vi "Load.vi"(8 "error in (no error)":errorcluster, 11 "Data File":path) -> (0 "error out":errorcluster, 3 "dup Data File":path)   [LabVIEW 2014, in "Map Data.lvlib"]
doc: "Loads data into the address book data store from a file on disk. If the file does not exist, the data store is initialized to being empty."
uses:
  Map Data.lvlib
  MapCommand.ctl
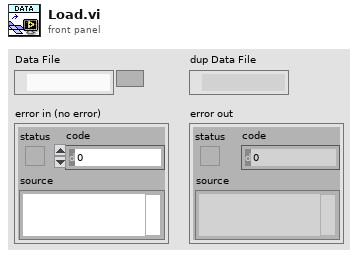
[diagram p1: front panel]
types:
  T1 = typedef "Map Data.lvlib/MapCommand.ctl" = enum16{"Load", "Update Cursor", "Save", "Get All Data", "Get Single Data", "Set Single Data", "Delete All", "Remove Single Data", "Set Favorite Status", "Is Data Modified", "Import Data"}
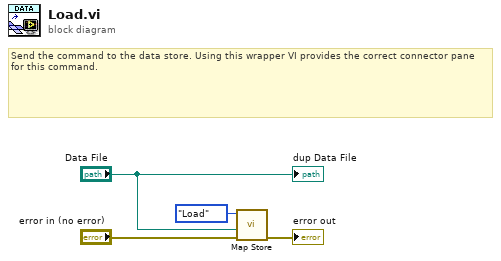
[diagram p0: block diagram]
diagram:
  # "Send the command to the data store. Using this wrapper VI provides the correct connector pane for this command."
  n1 = call "Map Store.vi"("error in (no error)"="error in (no error)", "Data File"="Data File", "Command"=MapCommand."Load") -> ("error out"=→"error out":errorcluster)  [unwired: 5 in, 3 out]
  "dup Data File" <- "Data File"
